vi "Handle Error.vi"(8 "error in (no error)":errorcluster, 11 "Application in":refnum<class "Application.lvclass">) -> (0 "error out":errorcluster, 2 "stop actor?":bool=TRUE, 3 "Application out":refnum<class "Application.lvclass">)   [LabVIEW 2020, in "Application.lvlib" / "Application.lvclass"]
doc: "(<B>Filename</B>: Actor Framework.lvlib:Actor.lvclass:Handle Error.vi)\n\nDefines how the actor handles an error that occurred while processing a message. By default, this method does nothing except stop the actor."
uses:
  Application.lvclass
  <vilib>/ActorFramework/Actor/Actor.lvclass
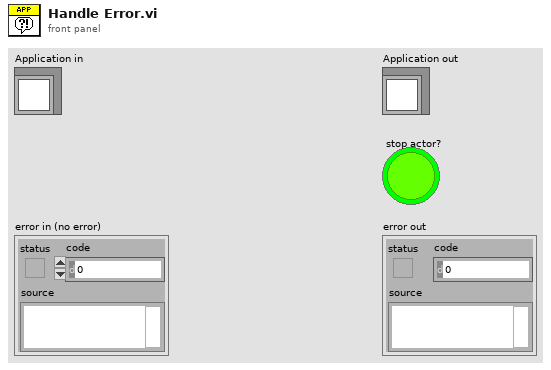
[diagram p1: front panel]
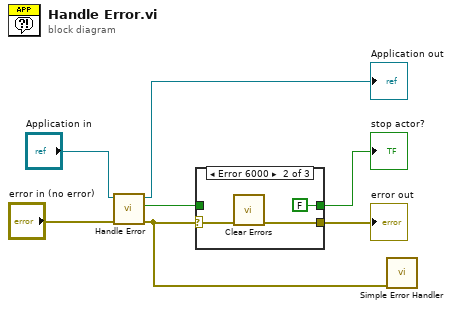
[diagram p0: block diagram]
diagram:
  n1 = call-parent "Handle Error.vi"("error in (no error)"="error in (no error)", "Actor in"="Application in") -> ("error out"=w4:errorcluster, "stop actor?"=w2:bool, "Actor out"=→"Application out":refnum<class "Application.lvclass">)  [unwired: 7 in]
  n2 = case shown="Error 6000" w4 {
    selector: w4 -> [w8 w11 w13]
    tunnel: [w9 FALSE ("stop actor?") w14] -> w3
    tunnel: w2 -> [w9 _ w14]
    tunnel: [w8 w10 w13] -> w1
    frame No Error {
    }
    frame Error {
      n3 = call <vilib>:"Clear Errors.vi"("error in (no error)"=w11) -> ("error out"=w10:errorcluster)  [unwired: 5 in, 1 out]
    }
    frame Default {
    }
  }
  "error out" <- w1
  "stop actor?" <- w3
  n4 = call <vilib>:"Simple Error Handler.vi"("error in (no error)"=w4) -> ()  [unwired: 4 in, 5 out]
